vi "Read Center Point.vi"(11 "StartOpenLoopScan in":refnum<class "StartOpenLoopScan.lvclass">) -> (2 "Center Point":dbl[unit], 3 "StartOpenLoopScan out":refnum<class "StartOpenLoopScan.lvclass">)   [LabVIEW 2015, in "StartOpenLoopScan.lvclass"]
uses:
  StartOpenLoopScan.lvclass
  StartOpenLoopScan.lvclass/StartOpenLoopScan.ctl
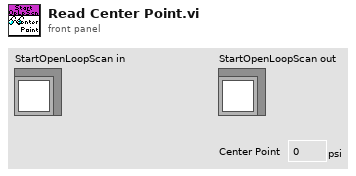
[diagram p1: front panel]
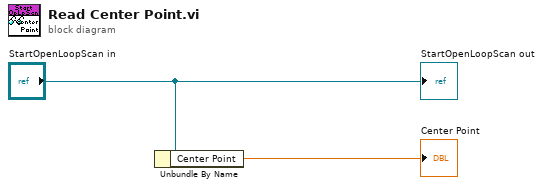
[diagram p0: block diagram]
diagram:
  n1 = Unbundle By Name("StartOpenLoopScan in") -> ("Center Point"=→"Center Point":dbl[unit])
  "StartOpenLoopScan out" <- "StartOpenLoopScan in"
